vi "Perform Action.vi"(8 "error in":errorcluster, 10 "Input":variant, 11 "Virt Instr Target in":refnum<class "Virt Instr Target.lvclass">) -> (0 "error out":errorcluster, 2 "Output":variant, 3 "Virt Instr Target out":refnum<class "Virt Instr Target.lvclass">)   [LabVIEW 2023, in "HAL GOOP4.lvlib" / "Virt Instr Target.lvclass"]
uses:
  Virt Instr Target.lvclass
  Virt Instr Target.lvclass/Virt Instr Target.ctl
  MSS Target/IMSS Target Actor Messages/Perform Action Msg/Perform Action Msg.lvclass
  Virt Instr Base/Virt Instr Base.lvclass
  <vilib>/ActorFramework/Message Enqueuer/Message Enqueuer.lvclass
  D:/git/HAL/HAL GOOP4/Virt Instr Host/Virt Instr Host.lvclass
  D:/git/HAL/HAL GOOP4/Virt Instr Base/Virt Instr Base.lvclass
  D:/git/HAL/HAL GOOP4/Virt Instr Target/Virt Instr Target.lvclass
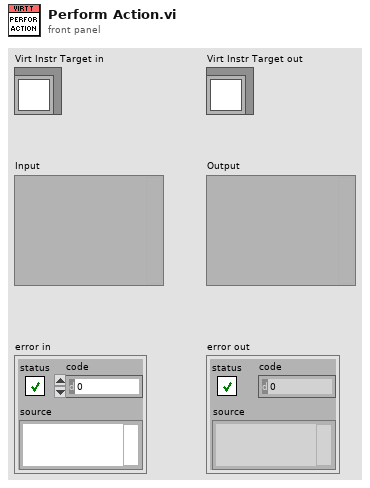
[diagram p1: front panel]
types:
  T1 = cluster{"MSS Target Enq":refnum<class "Message Enqueuer.lvclass">, "Point ident":string, "Data":variant}
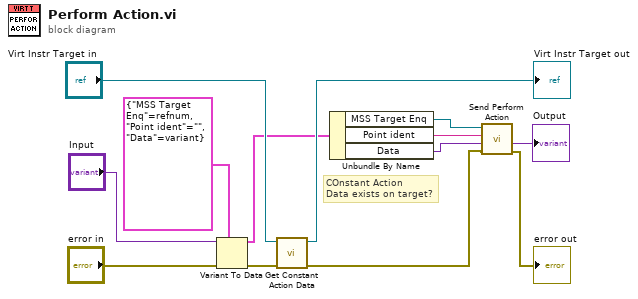
[diagram p0: block diagram]
diagram:
  # "COnstant Action\nData exists on target?"
  n1 = Variant To Data(error in="error in", type=T1 {"MSS Target Enq"=refnum, "Point ident"="", "Data"=variant}, Variant="Input") -> (data=w4:T1, error out=w9:errorcluster)
  n2 = call "Get Constant Action Data.vi"("error in (no error)"=w9, "Virt Instr Base in"="Virt Instr Target in") -> ("error out"=w13:errorcluster, "Virt Instr Base out"=→"Virt Instr Target out":refnum<class "Virt Instr Target.lvclass">)  [unwired: 7 in, 1 out]
  n3 = Unbundle By Name(w4) -> ("MSS Target Enq"=w3:refnum<class "Message Enqueuer.lvclass">, "Point ident"=w2:string, "Data"=w1:variant)
  n4 = call "Send Perform Action.vi"("error in"=w13, "Input"=w1, "Point Ident"=w2, "Message Enqueuer"=w3) -> ("error out"=→"error out":errorcluster, "Output"=→"Output":variant)  [unwired: 5 in, 1 out]
